vi "DevelopersERRORDefault.vi"(8 "error in (no error)":errorcluster) -> (0 "error out":errorcluster)   [LabVIEW 2016]
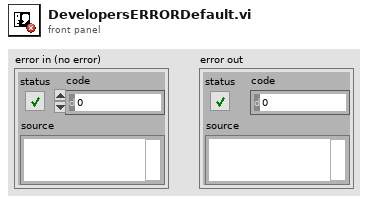
[diagram p1: front panel]
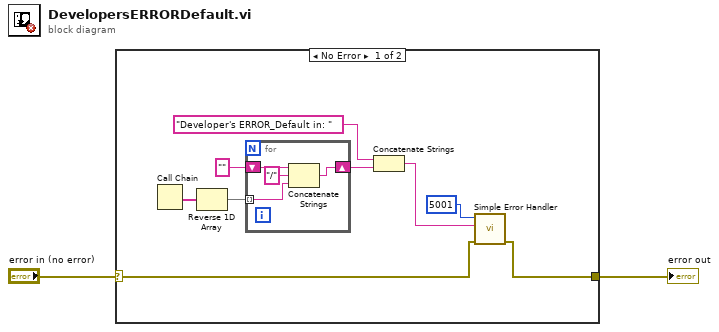
[diagram p0: block diagram]
diagram:
  n1 = case shown="No Error" "error in (no error)" {
    selector: "error in (no error)" -> [w3 w16]
    tunnel: [w11 w16] -> w1
    frame No Error {
      n2 = Call Chain() -> (call chain=w10:string[])
      n3 = Reverse 1D Array(array=w10) -> (reversed array=w9:string[])
      n4 = for {
        tunnel: w9 -> [w14] mode=indexing
        shift-right: [w12] -> w7
        shift-left: "" -> [w15]
        n5 = Concatenate Strings(w15, "/" ("string"), w14) -> (w12:string)
      }
      n6 = Concatenate Strings("Developer's ERROR_Default in: " ("string"), w7) -> (w5:string)
      n7 = call <vilib>:"Simple Error Handler.vi"("error code (no error:0)"=5001, "error source (\" \")"=w5, "error in (no error)"=w3) -> ("error out"=w11:errorcluster)  [unwired: 2 in, 4 out]
    }
    frame Error {
    }
  }
  "error out" <- w1
